vi "总磷总氮公式读取.vi"(8 "error in (no error)":errorcluster caption="错误输入（无错误）", 9 "量程":enum16{"低量程", "高量程"}(ring), 10 "测量模式":T1(ring), 11 "测量参数":u16(ring) items=["COD"=22, "氨氮"=3, "总氮"=2, "总磷"=1]) -> (0 "error out":errorcluster caption="错误输出", 3 "公式":cluster{"X^2":dbl, "X":dbl, "b":dbl})   [LabVIEW 2016, in "斯坦道CODCr.lvlib"]
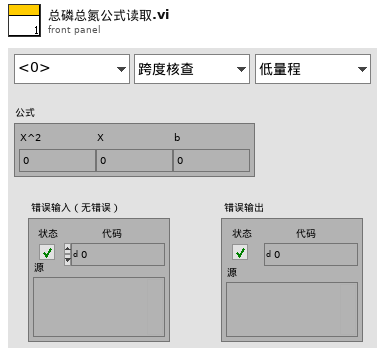
[diagram p1: front panel]
types:
  T1 = enum16{"跨度核查", "水样测量", "零点核查", "标样核查", "加标回收", "快捷测试", "空白校准", "标样校准"}
  T2 = cluster{"FLOAT[0]":sgl, "FLOAT[1]":sgl, "FLOAT[2]":sgl}
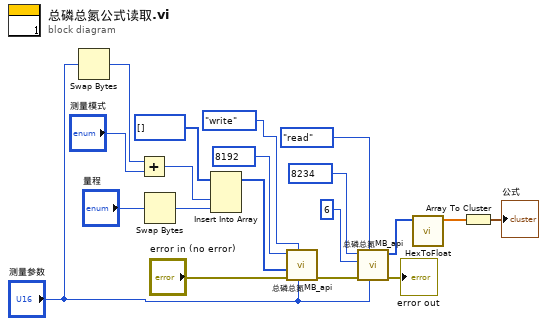
[diagram p0: block diagram]
diagram:
  n1 = Swap Bytes(anything="测量参数") -> (byte swapped=w4:u16)
  n2 = Add(x=w4, y="测量模式") -> (x+y=w12:u16)
  n3 = Swap Bytes(anything="量程") -> (byte swapped=w2:u16)
  n4 = Insert Into Array(array=u16[] [] ("数组"), new element #1=w12, new element #2=w2) -> (w6:u16[])  [unwired: 1 in]
  n5 = call "总磷总氮MB_api.vi"("Slave ID"="测量参数", "STEP"=enum16{"open", "read", "write", "close"}."write", "Error in"="error in (no error)", "values"=w6, "starting address"=u16 8192) -> ("error out"=w9:errorcluster)  [unwired: 4 in, 2 out]
  n6 = call "总磷总氮MB_api.vi"("Slave ID"="测量参数", "STEP"=enum16{"open", "read", "write", "close"}."read", "Error in"=w9, "quantity"=u16 6, "starting address"=u16 8234) -> ("error out"=→"error out":errorcluster, "Registers"=w18:u16[])  [unwired: 4 in, 1 out]
  n7 = call "HexToFloat.vi"("数组"=w18) -> ("FLOAT"=w17:sgl[])  [unwired: 10 in]
  n8 = Array To Cluster(array=w17) -> (cluster=→"公式":T2)
